vi "ZPL Config Output ON-OFF.vi"(6 "Settle (1 mS)":u32=1, 8 "error":errorcluster, 10 "Output ON":bool, 11 "VISA":refnum<visa-resource-name>) -> (0 "error out":errorcluster, 3 "VISA out":refnum<visa-resource-name>)   [LabVIEW 2016]
doc: "This VI sets the power supply output ON or OFF. No other settings change.\nIf \"Output ON\" is set FALSE, the output will be turned OFF.\n\nThis VI will wait for \"Settle\" milliseconds after setting the output. If unwired, there will be no delay"
panel:
  # "Lambda ZPLUS \n Serial Port\n  DC Power Supplies"
  # "Set the Output ON or OFF"
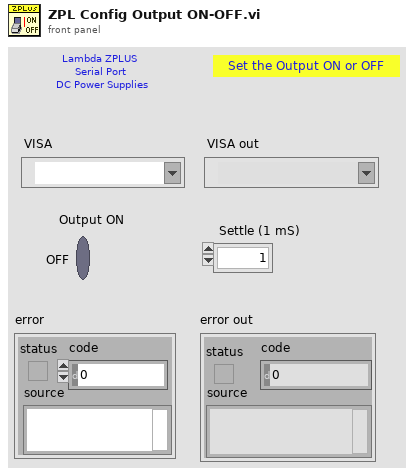
[diagram p1: front panel]
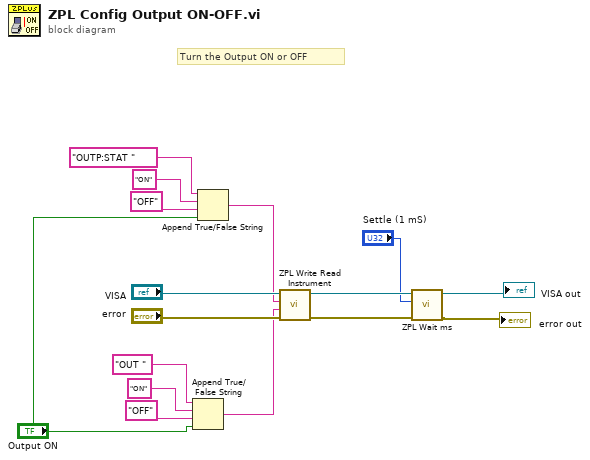
[diagram p0: block diagram]
diagram:
  # "Turn the Output ON or OFF"
  n1 = Append True/False String(1:"Output ON", 2:"OFF" ("format string"), 3:"ON" ("format string"), 4:"OUT " ("format string")) -> (0:w2:string)
  n2 = Append True/False String(1:"Output ON", 2:"OFF" ("format string"), 3:"ON" ("format string"), 4:"OUTP:STAT " ("format string")) -> (0:w8:string)
  n3 = call "ZPL Write Read Instrument.vi"("error in"="error", "Write Command/Query GEN"=w2, "Write Command/Query SCPI"=w8, "VISA"="VISA") -> ("error out"=w13:errorcluster, "VISA  out"=w14:refnum<visa-resource-name>)  [unwired: 5 in, 1 out]
  n4 = call "ZPL Wait ms.vi"("error"=w13, "Delay (1 mS)"="Settle (1 mS)", "VISA"=w14) -> ("error out"=→"error out":errorcluster, "VISA out"=→"VISA out":refnum<visa-resource-name>)  [unwired: 7 in]
